vi "Create.vi"(8 "error in (no error)":errorcluster, 9 "Create if not Found? (T)":bool=TRUE, 11 "User Event Name (\"\"=Unnamed)":string) -> (0 "error out":errorcluster, 1 "Created New?":bool, 2 "Is Registered?":bool, 3 "User Event":refnum<user-event>)   [LabVIEW 2018, in "UserEvent.lvlib"]
uses:
  UserEvent.lvlib
  <vilib>/Utility/error.llb/Error Cluster From Error Code.vi
  <vilib>/ErrorRing/Error Ring.xnode
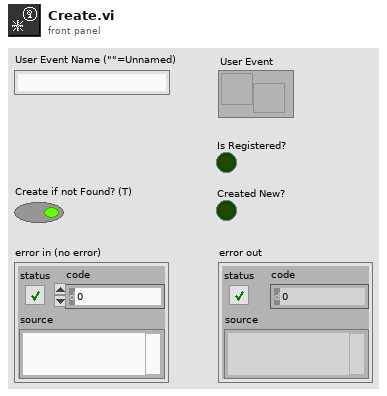
[diagram p1: front panel]
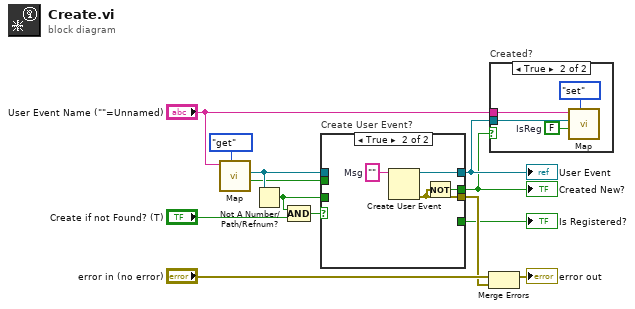
[diagram p0: block diagram]
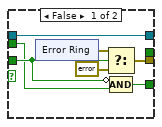
[diagram p2: hidden frame]
diagram:
  n1 = call "Map.vi"("Action"=enum8{"noop", "get", "set", "pop"}."get", "User Event Name"="User Event Name (\"\"=Unnamed)") -> ("Is Registered out"=w2:bool, "User Event out"=w6:refnum<user-event>)  [unwired: 7 in, 1 out]
  n2 = Not A Number/Path/Refnum?(number/path/refnum=w6) -> (NaN/Path/Refnum?=w3:bool)
  n3 = Compound Arithmetic op=AND(w3, "Create if not Found? (T)") -> (w10:bool)
  n4 = case "Create User Event?" shown="True" w10 {
    tunnel: [w17 w26] -> w7
    tunnel: [w20 w27] -> w5
    tunnel: [_ w25] -> w4
    tunnel: w6 -> [w20 _]
    tunnel: w3 -> [w16 _]
    tunnel: w2 -> [w15 _]
    tunnel: [w14 _] -> w1
    frame False {
      n5 = xnode "Error Ring"() -> ("error out"=w19:errorcluster)
      n6 = Select(t=w19, s=w16, f=errorcluster {"status"=FALSE, "code"=0, "source"=""}) -> (s? t:f=w17:errorcluster)
      n7 = Compound Arithmetic op=AND(invert w16, w15) -> (w14:bool)
    }
    frame True {
      w28 = ""  # Msg
      n8 = Create User Event(user event datatype=w28) -> (user event=w27:refnum<user-event>, error out=w26:errorcluster)  [unwired: 1 in]
      n9 = Not(x=w26) -> (.not. x?=w25:bool)
    }
  }
  "User Event" <- w5
  "Created New?" <- w4
  "Is Registered?" <- w1
  n10 = Merge Errors("error in (no error)", w7) -> (→"error out":errorcluster)
  n11 = case "Created?" shown="True" w4 {
    tunnel: "User Event Name (\"\"=Unnamed)" -> [_ w31]
    tunnel: w5 -> [_ w30]
    frame False {
    }
    frame True {
      w29 = FALSE  # IsReg
      n12 = call "Map.vi"("Action"=enum8{"noop", "get", "set", "pop"}."set", "Is Registered in"=w29, "User Event in"=w30, "User Event Name"=w31) -> ()  [unwired: 5 in, 3 out]
    }
  }
